vi "oa_Regulate Even Angle Signal (1 Channel).vi"(7 "reset?":bool, 8 "samples/rev":dbl, 9 "offset":dbl, 10 "time stamps":dbl[](array[numeric]) format="%.2f", 11 "Data":dbl[](array[numeric]) format="%.2f") -> (0 "actual max order":dbl, 2 "even-angle position info":T1, 3 "even-angle signal":cluster{"r0":dbl, "dr":dbl, "Y":dbl[]}={"r0"=0.0, "dr"=1.0, "Y"=[]} {"r0" format="%.2p"; "dr" format="%.2p"; "Y" format="%.2f"})   [LabVIEW 2017, in "SoundVib_Resampling.lvlib"]
uses:
  <vilib>/addons/Sound and Vibration/Order Analysis/Resample Order Tracking/SoundVib_Resampling.lvlib
  <vilib>/addons/Sound and Vibration/Order Analysis/Misc/OAT Position Info.ctl
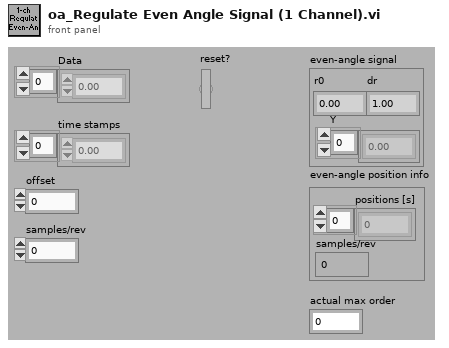
[diagram p1: front panel]
types:
  T1 = typedef "OAT Position Info.ctl" = cluster{"positions [s]":dbl[], "samples/rev":dbl}
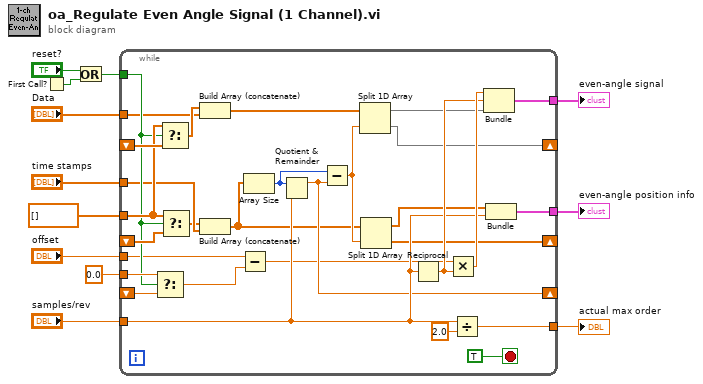
[diagram p0: block diagram]
diagram:
  n1 = First Call?() -> (First Call?: T/F=w5:bool)
  n2 = Or(x="reset?", y=w5) -> (x .or. y?=w6:bool)
  n3 = while {
    tunnel: "time stamps" -> [w28]
    tunnel: "offset" -> [w18]
    tunnel: "samples/rev" -> [w38]
    tunnel: "Data" -> [w29]
    shift-right: [w24] -> _
    shift-left: _ -> [w37]
    tunnel: dbl[] [] ("time stamps") -> [w35]
    tunnel: w6 -> [w32]
    shift-right: [w23] -> _
    shift-left: _ -> [w36]
    shift-right: [w20] -> _
    shift-left: _ -> [w34]
    tunnel: 0.0 ("t") -> [w33]
    tunnel: [w16] -> w3
    tunnel: [w15] -> w1
    tunnel: [w14] -> w2
    stop <- TRUE stop-if-true
    n4 = Select(t=w33, s=w32, f=w34) -> (s? t:f=w17:dbl)
    n5 = Select(t=w35, s=w32, f=w36) -> (s? t:f=w30:dbl[])
    n6 = Select(t=w35, s=w32, f=w37) -> (s? t:f=w27:dbl[])
    n7 = Build Array (concatenate)(w30, w29) -> (w25:dbl[])
    n8 = Build Array (concatenate)(w27, w28) -> (w13:dbl[])
    n9 = Subtract(x=w18, y=w17) -> (x-y=w19:dbl)
    n10 = Array Size(array=w13) -> (size(s)=w31:i32)
    n11 = Quotient & Remainder(x=w31, y=w38) -> (x-y*floor(x/y)=w20:dbl)  [unwired: 1 out]
    n12 = Subtract(x=w31, y=w20) -> (x-y=w26:dbl)
    n13 = Split 1D Array(array=w25, index=w26) -> (first subarray=w22:dbl[], second subarray=w23:dbl[])
    n14 = Split 1D Array(array=w13, index=w26) -> (first subarray=w21:dbl[], second subarray=w24:dbl[])
    n15 = Reciprocal(x=w38) -> (1/x=w41:dbl)
    n16 = Multiply(x=w19, y=w41) -> (x*y=w42:dbl)
    n17 = Divide(x=w38, y=2.0) -> (x/y=w14:dbl)
    n18 = Bundle(w42, w41, w22) -> (w16:cluster{dbl, dbl, dbl[]})  [unwired: 1 in]
    n19 = Bundle(w21, "samples/rev"=w38) -> (w15:cluster{dbl[], "samples/rev":dbl})  [unwired: 1 in]
  }
  "even-angle signal" <- w3
  "even-angle position info" <- w1
  "actual max order" <- w2
